vi "Generate_WayPoints_Hopping_Multi_CV.vi"(11 "Input Cluster":T2={"Scan Rate (um/s)"=15.0, "X Start"=15.0, "X End"=15.0, "Y Start"=15.0, "Y End"=15.0, " Z Start"=15.0, "HoppingDistance"=1.0, "Z End"=15.0, "Approach Rate Hopping (um/s)"=15.0, "Retrack Rate (um/s)"=15.0, "V 2"=15.0, "Approach Rate (um/s)"=15.0, "V 3"=15.0, "CV Rate / V/s"=15.0, "V 1"=15.0, "No. Cycles"=15.0}) -> (0 "output cluster":T1)   [LabVIEW 2023]
uses:
  TypeDefs/WayPointCluster.ctl
  User_Vi/Settings.vi
panel:
  in  "WayPointCluster":T1
  out "Y  P":dbl
  out "X  P":dbl
  out "HoppingDistanceX":dbl
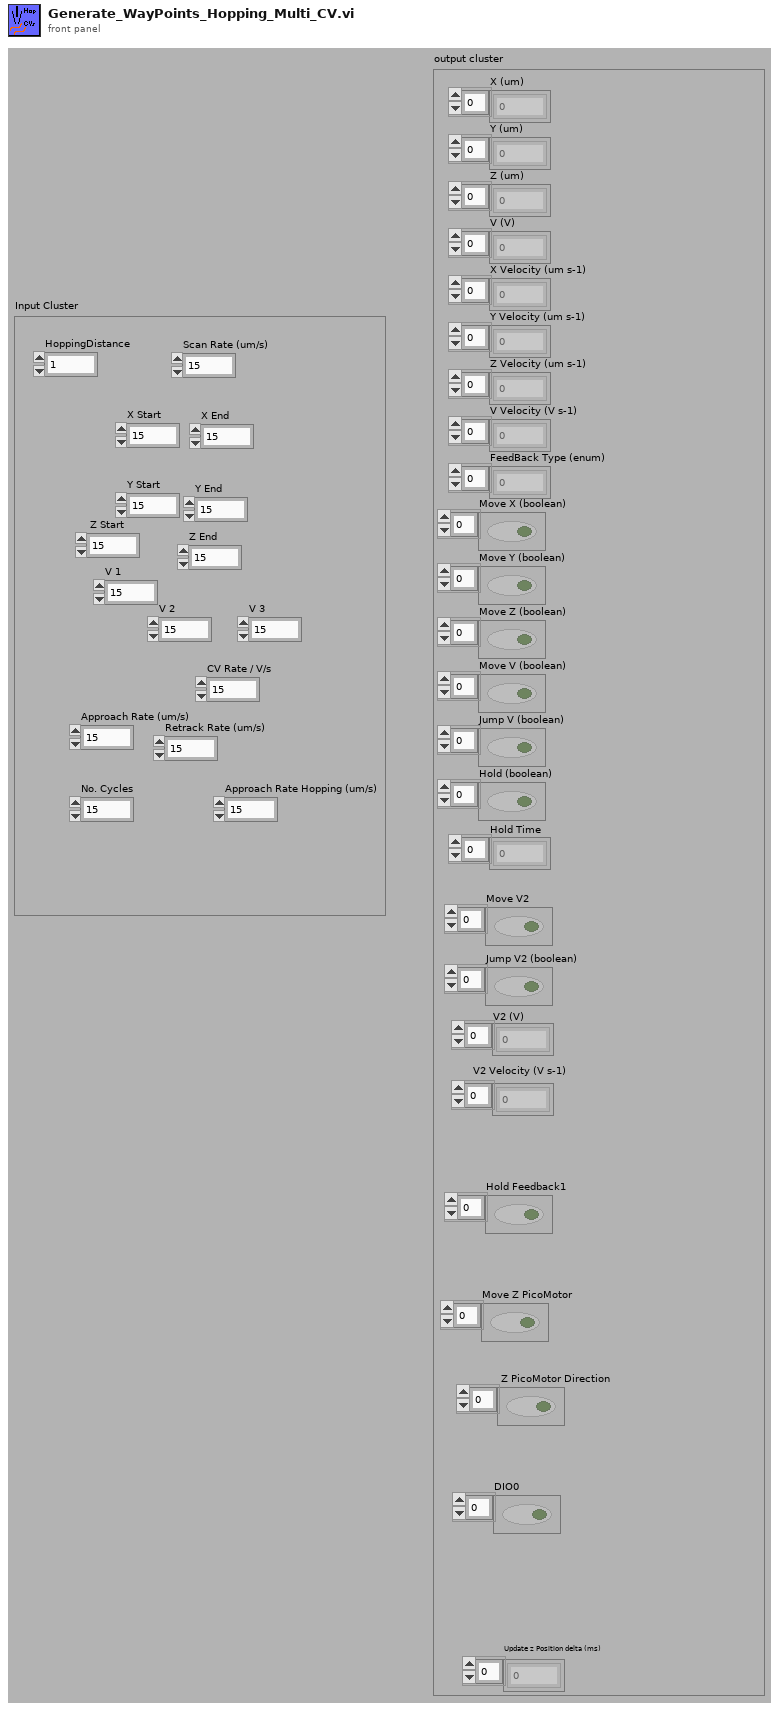
[diagram p1: front panel]
types:
  T1 = typedef "WayPointCluster.ctl" = cluster{"X (um)":dbl[], "Y (um)":dbl[], "Z (um)":dbl[], "V (V)":dbl[], "X Velocity (um s-1)":dbl[], "Y Velocity (um s-1)":dbl[], "Z Velocity (um s-1)":dbl[], "V Velocity (V s-1)":dbl[], "FeedBack Type (enum)":u16[], "Move X (boolean)":bool[], "Move Y (boolean)":bool[], "Move Z (boolean)":bool[], "Move V (boolean)":bool[], "Jump V (boolean)":bool[], "Hold (boolean)":bool[], "Hold Time":u32[], "V2 (V)":dbl[], "Move V2":bool[], "V2 Velocity (V s-1)":dbl[], "Jump V2 (boolean)":bool[], "Update z Position delta (ms)":i16[], "Hold Feedback1":bool[], "Move Z PicoMotor":bool[], " Z PicoMotor Direction":bool[], "DIO0":bool[]}
  T2 = cluster{"Scan Rate (um/s)":dbl, "X Start":dbl, "X End":dbl, "Y Start":dbl, "Y End":dbl, " Z Start":dbl, "HoppingDistance":dbl, "Z End":dbl, "Approach Rate Hopping (um/s)":dbl, "Retrack Rate (um/s)":dbl, "V 2":dbl, "Approach Rate (um/s)":dbl, "V 3":dbl, "CV Rate / V/s":dbl, "V 1":dbl, "No. Cycles":dbl}
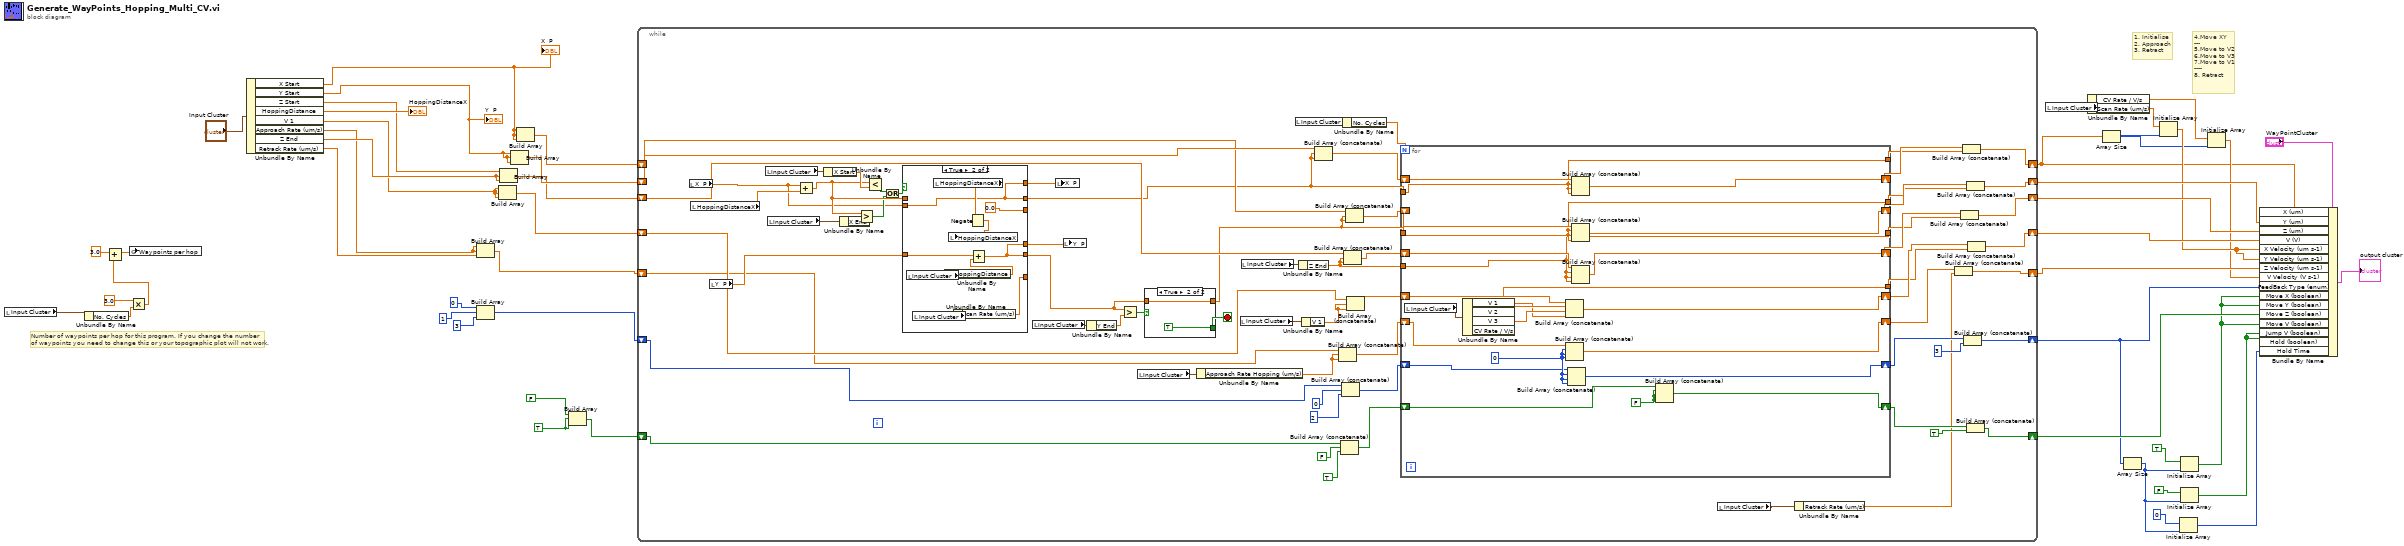
[diagram p0: block diagram]
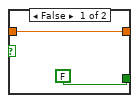
[diagram p2: hidden frame]
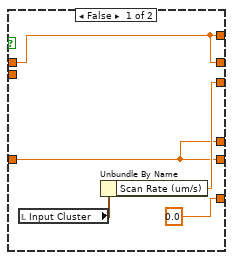
[diagram p3: hidden frame]
diagram:
  w8 = TRUE
  # "Number of waypoints per hop for this program. If you change the number\nof waypoints you need to change this or your topographic plot will not work."
  # "4.Move XY\n---\n5.Move to V2\n6.Move to V3\n7.Move to V1\n----\n8. Retract"
  # "1. Initialise\n2. Approach\n3. Retract"
  n1 = local read "Input Cluster"() -> (w5:T2)
  n2 = Unbundle By Name(w5) -> ("No. Cycles"=w3:dbl)
  n3 = Multiply(x=3.0, y=w3) -> (x*y=w1:dbl)
  n4 = Add(x=3.0, y=w1) -> (x+y=w4:dbl)
  n5 = global write "Settings.vi" "Waypoints per hop"(w4) -> ()
  n6 = Unbundle By Name("Input Cluster") -> ("X Start"=w35:dbl, "Y Start"=w34:dbl, "Z Start"=w36:dbl, "HoppingDistance"=→"HoppingDistanceX":dbl, "V 1"=w32:dbl, "Approach Rate (um/s)"=w27:dbl, "Z End"=w33:dbl, "Retrack Rate (um/s)"=w31:dbl)
  "X  P" <- w35
  "Y  P" <- w34
  n7 = Build Array(w27, w27, w31) -> (w40:dbl[])
  n8 = Build Array(u16 0 ("element"), u16 1 ("element"), u16 3 ("element")) -> (w38:u16[])
  n9 = Build Array(w32, w32, w32) -> (w42:dbl[])
  n10 = Build Array(w36, w33, w33) -> (w44:dbl[])
  n11 = Build Array(w34, w34, w34) -> (w46:dbl[])
  n12 = Build Array(w35, w35, w35) -> (w47:dbl[])
  n13 = Build Array(FALSE, w8, w8) -> (w24:bool[])
  n14 = while {
    shift-right: [w96] -> w17
    shift-left: w47 -> [w82]
    shift-right: [w93] -> w45
    shift-left: w46 -> [w80]
    shift-right: [w90] -> w43
    shift-left: w44 -> [w78]
    shift-right: [w87] -> w41
    shift-left: w42 -> [w76]
    shift-right: [w84] -> w39
    shift-left: w40 -> [w71]
    shift-right: [w70] -> w16
    shift-left: w38 -> [w57]
    shift-right: [w62] -> w29
    shift-left: w24 -> [w55]
    stop <- w105 stop-if-true
    n15 = local read "X  P"() -> (w104:dbl)
    n16 = local read "HoppingDistanceX"() -> (w115:dbl)
    n17 = local read "Y  P"() -> (w103:dbl)
    n18 = local read "Input Cluster"() -> (w117:T2)
    n19 = local read "Input Cluster"() -> (w116:T2)
    n20 = Add(x=w104, y=w115) -> (x+y=w111:dbl)
    n21 = Unbundle By Name(w117) -> ("X Start"=w114:dbl)
    n22 = Unbundle By Name(w116) -> ("X End"=w112:dbl)
    n23 = Greater?(x=w111, y=w112) -> (0:w110:bool)
    n24 = Less?(x=w111, y=w114) -> (x < y?=w113:bool)
    n25 = Or(x=w113, y=w110) -> (x .or. y?=w109:bool)
    n26 = case shown="True" w109 {
      tunnel: w111 -> [w145 _]
      tunnel: [w145 w151] -> w67
      tunnel: w104 -> [_ w151]
      tunnel: w103 -> [w146 w152]
      tunnel: [w146 w150] -> w102
      tunnel: [w148 0.0] -> _
      tunnel: [0.0 w153] -> _
      tunnel: [w146 w150] -> w101
      tunnel: [w145 w151] -> w100
      frame False {
        n27 = local read "Input Cluster"() -> (w149:T2)
        n28 = Unbundle By Name(w149) -> ("Scan Rate (um/s)"=w148:dbl)
      }
      frame True {
        n29 = local read "Input Cluster"() -> (w157:T2)
        n30 = local read "Input Cluster"() -> (w155:T2)
        n31 = local read "HoppingDistanceX"() -> (w159:dbl)
        n32 = Unbundle By Name(w157) -> ("HoppingDistance"=w156:dbl)
        n33 = Unbundle By Name(w155) -> ("Scan Rate (um/s)"=w153:dbl)
        n34 = Negate(x=w159) -> (-x=w158:dbl)
        n35 = local write "HoppingDistanceX"(w158) -> ()
        n36 = Add(x=w152, y=w156) -> (x+y=w150:dbl)
      }
    }
    n37 = local read "Input Cluster"() -> (w108:T2)
    n38 = local write "X  P"(w100) -> ()
    n39 = local write "Y  P"(w101) -> ()
    n40 = Unbundle By Name(w108) -> ("Y End"=w107:dbl)
    n41 = Greater?(x=w102, y=w107) -> (0:w106:bool)
    n42 = local read "Input Cluster"() -> (w99:T2)
    n43 = case shown="True" w106 {
      tunnel: w102 -> [w142 w144]
      tunnel: [w142 w144] -> w66
      tunnel: [FALSE TRUE] -> w105
      frame False {
      }
      frame True {
      }
    }
    n44 = Unbundle By Name(w99) -> ("Approach Rate Hopping (um/s)"=w63:dbl)
    n45 = local read "Input Cluster"() -> (w75:T2)
    n46 = local read "Input Cluster"() -> (w77:T2)
    n47 = local read "Input Cluster"() -> (w98:T2)
    n48 = Unbundle By Name(w77) -> ("Z End"=w65:dbl)
    n49 = Unbundle By Name(w75) -> ("V 1"=w64:dbl)
    n50 = Build Array (concatenate)(w82, w67, w67) -> (w83:dbl[])
    n51 = Build Array (concatenate)(w71, w63, w63) -> (w72:dbl[])
    n52 = Build Array (concatenate)(w55, FALSE, TRUE) -> (w54:bool[])
    n53 = Build Array (concatenate)(w57, u16 0, u16 2) -> (w56:u16[])
    n54 = Unbundle By Name(w98) -> ("No. Cycles"=w97:dbl)
    n55 = Build Array (concatenate)(w78, w65, w65) -> (w79:dbl[])
    n56 = Build Array (concatenate)(w80, w66, w66) -> (w81:dbl[])
    n57 = Build Array (concatenate)(w76, w64, w64) -> (w74:dbl[])
    n58 = for {
      N: w97 -> [_]
      tunnel: w67 -> [w129]
      shift-right: [w138] -> w95
      shift-left: w83 -> [w139]
      shift-right: [w136] -> w92
      shift-left: w81 -> [w137]
      tunnel: w66 -> [w128]
      shift-right: [w134] -> w89
      shift-left: w79 -> [w135]
      shift-right: [w130] -> w86
      shift-left: w74 -> [w131]
      tunnel: [w129] -> w94
      tunnel: [w128] -> w91
      tunnel: [w126] -> w88
      tunnel: [w127] -> w85
      shift-right: [w124] -> w73
      shift-left: w72 -> [w125]
      tunnel: w65 -> [w126]
      shift-right: [w123] -> w69
      shift-left: w56 -> [w121]
      shift-right: [w120] -> w60
      shift-left: w54 -> [w119]
      w118 = FALSE
      w122 = u16 0
      n59 = local read "Input Cluster"() -> (w140:T2)
      n60 = Unbundle By Name(w140) -> ("V 1"=w127:dbl, "V 2"=w133:dbl, "V 3"=w132:dbl)  [unwired: 1 out]
      n61 = Build Array (concatenate)(w131, w133, w132, w127) -> (w130:dbl[])
      n62 = Build Array (concatenate)(w125, w122, w122, w122) -> (w124:dbl[])
      n63 = Build Array (concatenate)(w121, w122, w122, w122) -> (w123:u16[])
      n64 = Build Array (concatenate)(w139, w129, w129, w129) -> (w138:dbl[])
      n65 = Build Array (concatenate)(w137, w128, w128, w128) -> (w136:dbl[])
      n66 = Build Array (concatenate)(w135, w126, w126, w126) -> (w134:dbl[])
      n67 = Build Array (concatenate)(w119, w118, w118, w118) -> (w120:bool[])
    }
    n68 = local read "Input Cluster"() -> (w59:T2)
    n69 = Unbundle By Name(w59) -> ("Retrack Rate (um/s)"=w58:dbl)
    n70 = Build Array (concatenate)(w73, w58) -> (w84:dbl[])
    n71 = Build Array (concatenate)(w89, w88) -> (w90:dbl[])
    n72 = Build Array (concatenate)(w95, w94) -> (w96:dbl[])
    n73 = Build Array (concatenate)(w69, u16 3) -> (w70:u16[])
    n74 = Build Array (concatenate)(w60, TRUE) -> (w62:bool[])
    n75 = Build Array (concatenate)(w92, w91) -> (w93:dbl[])
    n76 = Build Array (concatenate)(w86, w85) -> (w87:dbl[])
  }
  n77 = local read "Input Cluster"() -> (w23:T2)
  n78 = Unbundle By Name(w23) -> ("CV Rate / V/s"=w20:dbl, "Scan Rate (um/s)"=w22:dbl)
  n79 = Array Size(array=w17) -> (size(s)=w19:i32)
  n80 = Array Size(array=w16) -> (size(s)=w12:i32)
  n81 = Initialize Array(w22, w19) -> (w21:dbl[])
  n82 = Initialize Array(u16 0, w12) -> (w10:u16[])
  n83 = Initialize Array(TRUE, w12) -> (w14:bool[])
  n84 = Initialize Array(FALSE, w12) -> (w7:bool[])
  n85 = Initialize Array(w20, w19) -> (w18:dbl[])
  n86 = Bundle By Name(cluster="WayPointCluster", "X (um)"=w17, "Y (um)"=w45, "Z (um)"=w43, "V (V)"=w41, "X Velocity (um s-1)"=w21, "Y Velocity (um s-1)"=w21, "Z Velocity (um s-1)"=w39, "V Velocity (V s-1)"=w18, "FeedBack Type (enum)"=w16, "Move X (boolean)"=w14, "Move Y (boolean)"=w14, "Move Z (boolean)"=w29, "Move V (boolean)"=w14, "Jump V (boolean)"=w7, "Hold (boolean)"=w7, "Hold Time"=w10) -> (→"output cluster":T1)
